vi "ReadADC_NB.vi"(6 "error in (no error)":errorcluster, 9 "ADC to Read":string(combo)="VA") -> (0 "error out":errorcluster, 3 "ADC Value Read":dbl)   [LabVIEW 2011]
doc: "This VI reads a chosen ADC value from the NB PLL instance.\n\nInputs:\n1. ADC to Read: Selects the ADC that will be read through JTAG (ie. LVL, VA, VD, etc.).\n\nOutputs:\n1.ADC Value Read: The value of the chosen ADC in binary."
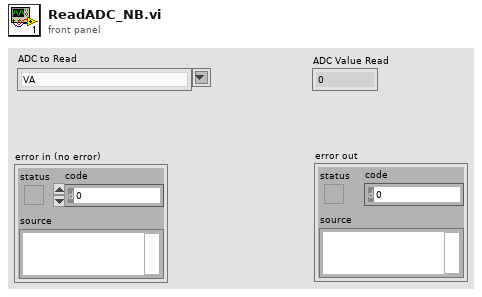
[diagram p1: front panel]
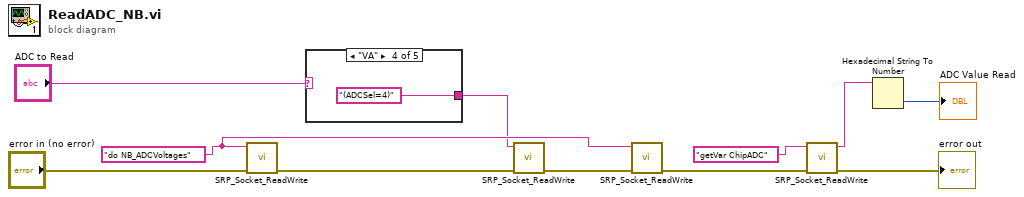
[diagram p0: block diagram]
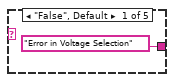
[diagram p2: hidden frame]
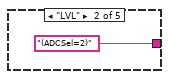
[diagram p3: hidden frame]
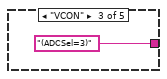
[diagram p4: hidden frame]
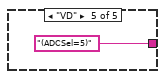
[diagram p5: hidden frame]
diagram:
  w5 = "do NB_ADCVoltages"
  n1 = call "SRP_Socket_ReadWrite.vi"("error in (no error)"="error in (no error)", "Data In"=w5) -> ("error out"=w8:errorcluster)  [unwired: 7 in, 1 out]
  n2 = case shown="\"VA\"" "ADC to Read" {
    tunnel: ["Error in Voltage Selection" "(ADCSel=2)" "(ADCSel=3)" "(ADCSel=4)" "(ADCSel=5)"] -> w4
    frame "False", Default {
    }
    frame "LVL" {
    }
    frame "VCON" {
    }
    frame "VA" {
    }
    frame "VD" {
    }
  }
  n3 = call "SRP_Socket_ReadWrite.vi"("error in (no error)"=w8, "Data In"=w4) -> ("error out"=w7:errorcluster)  [unwired: 7 in, 1 out]
  n4 = call "SRP_Socket_ReadWrite.vi"("error in (no error)"=w7, "Data In"=w5) -> ("error out"=w6:errorcluster)  [unwired: 7 in, 1 out]
  n5 = call "SRP_Socket_ReadWrite.vi"("error in (no error)"=w6, "Data In"="getVar ChipADC") -> ("error out"=→"error out":errorcluster, "Data Out"=w2:string)  [unwired: 7 in]
  n6 = Hexadecimal String To Number(string=w2) -> (number=→"ADC Value Read":u32)  [unwired: 2 in, 1 out]
